vi "Desafio Ford.vi"() -> ()   [LabVIEW 2018]
panel:
  in  "file path (use dialog)":path
  out "Resultado":string[](array[string])
  out "Notas":string[](array[string])
  out "Gabarito":string
  out "Pontos":i32[](array[numeric])
  in  "data.txt":string[](array[string])
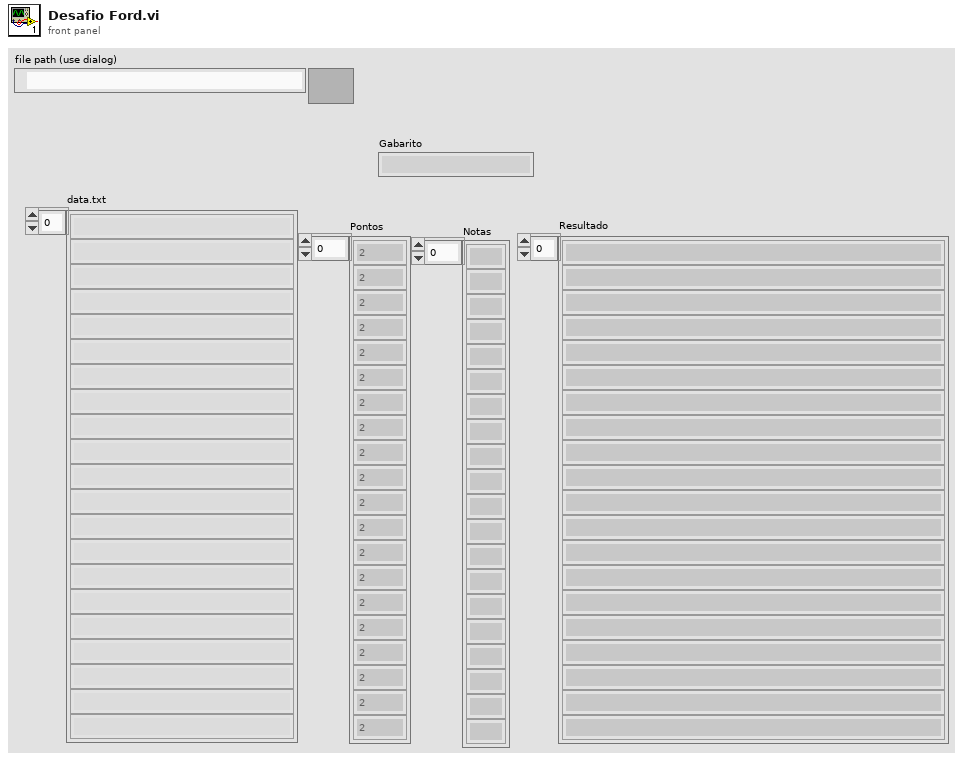
[diagram p1: front panel]
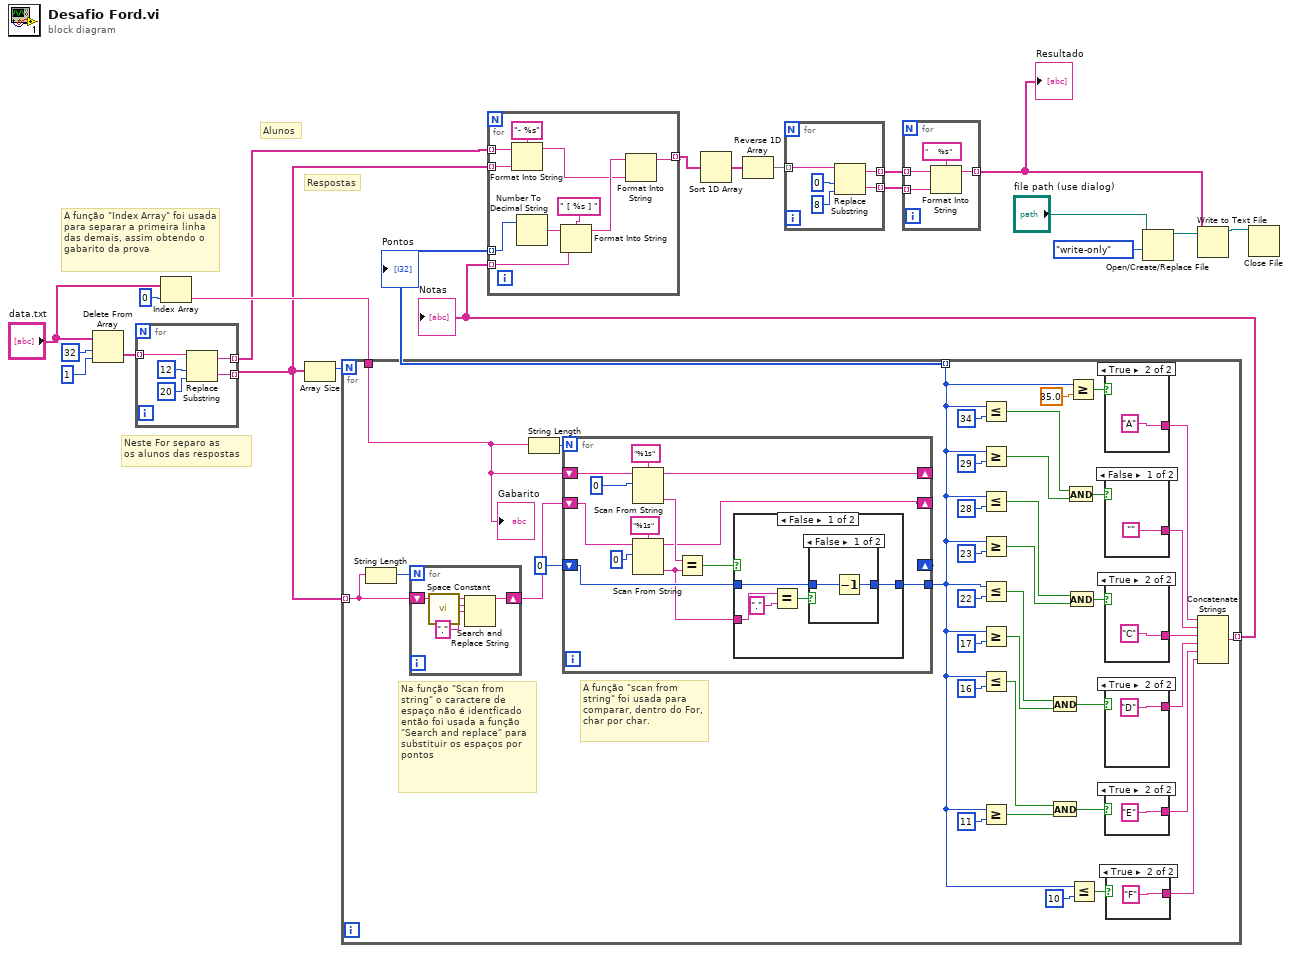
[diagram p0: block diagram]
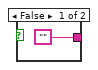
[diagram p2: hidden frame]
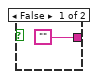
[diagram p3: hidden frame]
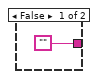
[diagram p4: hidden frame]
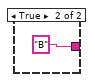
[diagram p5: hidden frame]
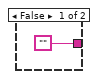
[diagram p6: hidden frame]
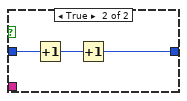
[diagram p8: hidden frame]
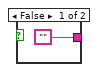
[diagram p9: hidden frame]
diagram:
  # "Respostas"
  # "Alunos"
  # "A função \"Index Array\" foi usada para separar a primeira linha das demais, assim obtendo o gabarito da prova"
  # "Neste For separo as \nos alunos das respostas"
  n1 = Delete From Array(array="data.txt", length=32, index=1) -> (deleted portion=w16:string[])  [unwired: 1 out]
  n2 = for {
    tunnel: w16 -> [w22] mode=indexing
    tunnel: [w24] -> w13 mode=indexing
    tunnel: [w23] -> w14 mode=indexing
    n3 = Replace Substring(2:20 ("length"), 3:12 ("offset (0)"), 5:w22) -> (0:w24:string, 1:w23:string)  [unwired: 1 in]
  }
  n4 = Index Array(array="data.txt", index=0) -> (element=w20:string)
  n5 = Array Size(array=w13) -> (size(s)=w15:i32)
  n6 = for {
    N: w15 -> [_]
    tunnel: w20 -> [w36]
    tunnel: [w29] -> w12 mode=indexing
    tunnel: [w28] -> w11 mode=indexing
    tunnel: w13 -> [w27] mode=indexing
    # "A função \"scan from string\" foi usada para comparar, dentro do For, char por char."
    # "Na função \"Scan from\nstring\" o caractere de\nespaço não é identficado\nentão foi usada a função \n\"Search and replace\" para substituir os espaços por pontos"
    n7 = String Length(string=w27) -> (length=w62:i32)
    n8 = for {
      N: w62 -> [_]
      shift-right: [w76] -> w61
      shift-left: w27 -> [w75]
      n9 = call <vilib>:"Space Constant.vi"() -> ("String"=w77:string)
      n10 = Search and Replace String(input string=w75, search string=w77, replace string=".") -> (result string=w76:string)  [unwired: 5 in, 3 out]
    }
    n11 = String Length(string=w36) -> (length=w63:i32)
    n12 = for {
      N: w63 -> [_]
      shift-right: [w79] -> _
      shift-left: 0 -> [w90]
      shift-right: [w81] -> _
      shift-left: w36 -> [w83]
      shift-right: [w80] -> _
      shift-left: w61 -> [w82]
      tunnel: [w79] -> w28
      n13 = Scan From String(format string="%1s", input string=w83, initial scan location=u32 0) -> (remaining string=w81:string, output 1=w84:string)  [unwired: 2 in, 2 out]
      n14 = Scan From String(format string="%1s", input string=w82, initial scan location=u32 0) -> (remaining string=w80:string, output 1=w87:string)  [unwired: 2 in, 2 out]
      n15 = Equal?(x=w84, y=w87) -> (x = y?=w91:bool)
      n16 = case shown="False" w91 {
        tunnel: [w94 w101] -> w79
        tunnel: w90 -> [w95 w100]
        tunnel: w87 -> [w92 _]
        frame False {
          n17 = Equal?(x=w92, y="." ("String")) -> (x = y?=w96:bool)
          n18 = case shown="False" w96 {
            tunnel: w95 -> [w98 w99]
            tunnel: [w97 w99] -> w94
            frame False {
              n19 = Decrement(x=w98) -> (x-1=w97:i32)
            }
            frame True {
            }
          }
        }
        frame True {
          n20 = Increment(x=w100) -> (x+1=w102:i32)
          n21 = Increment(x=w102) -> (x+1=w101:i32)
        }
      }
    }
    n22 = Less Or Equal?(x=w28, y=34) -> (x <= y?=w59:bool)
    n23 = Greater Or Equal?(x=w28, y=29) -> (x >= y?=w57:bool)
    n24 = Less Or Equal?(x=w28, y=28) -> (x <= y?=w53:bool)
    n25 = Greater Or Equal?(x=w28, y=23) -> (x >= y?=w51:bool)
    n26 = Less Or Equal?(x=w28, y=22) -> (x <= y?=w48:bool)
    n27 = Greater Or Equal?(x=w28, y=17) -> (x >= y?=w46:bool)
    n28 = Less Or Equal?(x=w28, y=16) -> (x <= y?=w43:bool)
    n29 = Greater Or Equal?(x=w28, y=11) -> (x >= y?=w41:bool)
    n30 = And(x=w48, y=w46) -> (x .and. y?=w44:bool)
    n31 = And(x=w43, y=w41) -> (x .and. y?=w39:bool)
    n32 = And(x=w59, y=w57) -> (x .and. y?=w54:bool)
    n33 = And(x=w53, y=w51) -> (x .and. y?=w49:bool)
    n34 = Greater Or Equal?(x=w28, y=35.0) -> (x >= y?=w55:bool)
    n35 = Less Or Equal?(x=w28, y=10) -> (x <= y?=w37:bool)
    n36 = case shown="True" w55 {
      tunnel: ["" "A"] -> w35
      frame False {
      }
      frame True {
      }
    }
    n37 = case shown="False" w54 {
      tunnel: ["" "B"] -> w34
      frame False {
      }
      frame True {
      }
    }
    n38 = case shown="True" w49 {
      tunnel: ["" "C"] -> w33
      frame False {
      }
      frame True {
      }
    }
    n39 = case shown="True" w44 {
      tunnel: ["" "D"] -> w32
      frame False {
      }
      frame True {
      }
    }
    n40 = case shown="True" w39 {
      tunnel: ["" "E"] -> w31
      frame False {
      }
      frame True {
      }
    }
    n41 = case shown="True" w37 {
      tunnel: ["" "F"] -> w30
      frame False {
      }
      frame True {
      }
    }
    n42 = Concatenate Strings(w35, w34, w33, w32, w31, w30) -> (w29:string)
    "Gabarito" <- w36
  }
  "Notas" <- w12
  "Pontos" <- w11
  n43 = for {
    tunnel: w14 -> [w114] mode=indexing
    tunnel: w13 -> [w112] mode=indexing
    tunnel: w12 -> [w108] mode=indexing
    tunnel: w11 -> [w110] mode=indexing
    tunnel: [w107] -> w10 mode=indexing
    n44 = Format Into String(format string="- %s", initial string=w114, w112) -> (resulting string=w105:string)  [unwired: 1 in, 1 out]
    n45 = Number To Decimal String(number=w110) -> (decimal integer string=w109:string)  [unwired: 1 in]
    n46 = Format Into String(format string=" [ %s ] ", initial string=w109, w108) -> (resulting string=w106:string)  [unwired: 1 in, 1 out]
    n47 = Format Into String(initial string=w106, w105) -> (resulting string=w107:string)  [unwired: 2 in, 1 out]
  }
  n48 = Sort 1D Array(array=w10) -> (sorted array=w9:string[])
  n49 = Reverse 1D Array(array=w9) -> (reversed array=w8:string[])
  n50 = for {
    tunnel: w8 -> [w119] mode=indexing
    tunnel: [w117] -> w7 mode=indexing
    tunnel: [w118] -> w6 mode=indexing
    n51 = Replace Substring(2:8 ("length (len. of substring)"), 3:0 ("offset (0)"), 5:w119) -> (0:w117:string, 1:w118:string)  [unwired: 1 in]
  }
  n52 = for {
    tunnel: w7 -> [w122] mode=indexing
    tunnel: w6 -> [w121] mode=indexing
    tunnel: [w120] -> w3 mode=indexing
    n53 = Format Into String(format string="     %s", initial string=w121, w122) -> (resulting string=w120:string)  [unwired: 1 in, 1 out]
  }
  "Resultado" <- w3
  n54 = Open/Create/Replace File(file path (use dialog)="file path (use dialog)", access (0:read/write)=enum16{"read/write", "read-only", "write-only"}."write-only") -> (refnum out=w4:refnum<file>)  [unwired: 4 in, 2 out]
  n55 = Write to Text File(file (use dialog)=w4, text=w3) -> (refnum out=w2:refnum<file>)  [unwired: 2 in, 2 out]
  n56 = Close File(refnum=w2) -> ()  [unwired: 1 in, 2 out]
